vi "Logcluster Array to String Array.vi"(0 "UDcluster Array in":T1[](array[typedef]), 11 "error in (no error)":errorcluster) -> (4 "UDarray out":string[](array[string]), 15 "error out":errorcluster)   [LabVIEW 2012]
uses:
  typedef/Log_User_Data.ctl
  typedef/User Accounts.ctl
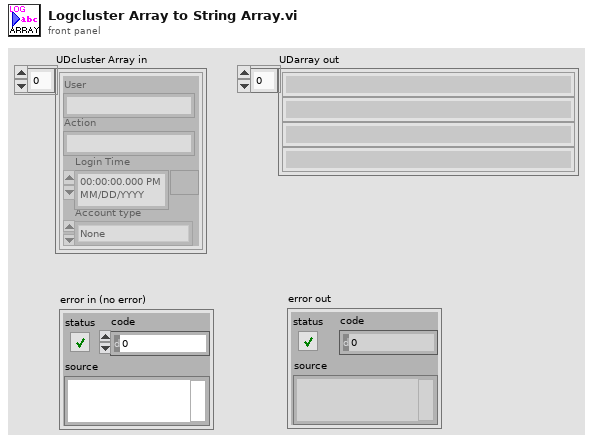
[diagram p1: front panel]
types:
  T1 = typedef "Log_User_Data.ctl" = cluster{"User":string, "Action":string, "Account type":T2, "Login Time ":timestamp}
  T2 = typedef "User Accounts.ctl" = enum16{"None", "User", "Admin"}
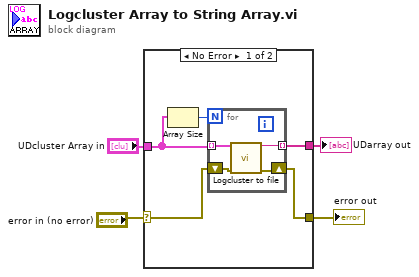
[diagram p0: block diagram]
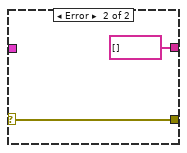
[diagram p2: hidden frame]
diagram:
  n1 = case shown="No Error" "error in (no error)" {
    selector: "error in (no error)" -> [w5 w15]
    tunnel: [w9 string[] []] -> w4
    tunnel: "UDcluster Array in" -> [w8 _]
    tunnel: [w6 w15] -> w1
    frame No Error {
      n2 = Array Size(array=w8) -> (size(s)=w7:i32)
      n3 = for {
        N: w7 -> [_]
        tunnel: w8 -> [w13] mode=indexing
        tunnel: [w12] -> w9 mode=indexing
        shift-right: [w10] -> w6
        shift-left: w5 -> [w11]
        n4 = call "Logcluster to file.vi"("Log Cluster"=w13, "error in (no error)"=w11) -> ("CypheredText"=w12:string, "error out"=w10:errorcluster)  [unwired: 12 in]
      }
    }
    frame Error {
    }
  }
  "UDarray out" <- w4
  "error out" <- w1
